vi "_ObtainQueue.vi"(5 "MessageQueue Type":refnum<class "MessageQueue.lvclass">, 7 "Max Queue Size (-1, unlimited)":i32=-1, 8 "error in (no error)":errorcluster, 10 "Create if Not Found? (T)":bool=TRUE, 11 "Queue Name":string) -> (0 "error out":errorcluster, 1 "Created New?":bool, 3 "MessageQueue out":refnum<class "MessageQueue.lvclass">)   [LabVIEW 2013, in "LapDog.Messaging.v3.lvlib" / "MessageQueue.lvclass"]
doc: "Creates a MessageQueue object. \n\nChild classes should use this method in their creator method, passing a child class object in on the MessageQueue Type terminal."
uses:
  MessageQueue.lvclass
  Message/Message.lvclass
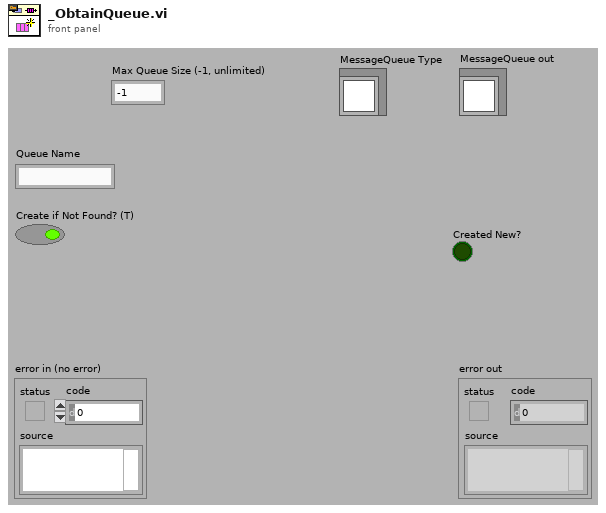
[diagram p1: front panel]
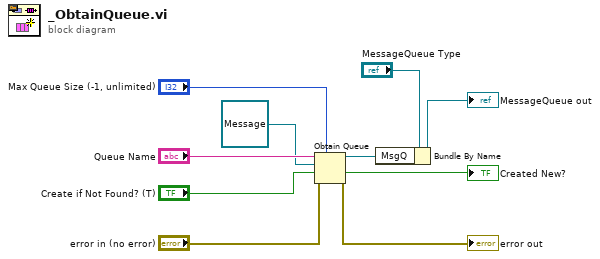
[diagram p0: block diagram]
diagram:
  n1 = Obtain Queue(max queue size (-1, unlimited)="Max Queue Size (-1, unlimited)", name (unnamed)="Queue Name", element data type=refnum<class "Message.lvclass"> refnum ("MessageLibrary.lvlib:Message"), create if not found? (T)="Create if Not Found? (T)", error in (no error)="error in (no error)") -> (queue out=w2:refnum<queue>, created new?=→"Created New?":bool, error out=→"error out":errorcluster)
  n2 = Bundle By Name(cluster="MessageQueue Type", "MsgQ"=w2) -> (→"MessageQueue out":refnum<class "MessageQueue.lvclass">)
